vi "timerRun.vi"() -> ()   [LabVIEW 2012]
panel:
  in  "stop":bool
  out "Run time":timestamp
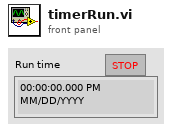
[diagram p1: front panel]
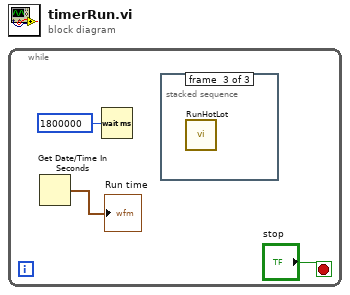
[diagram p0: block diagram]
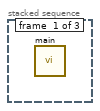
[diagram p2: hidden frame]
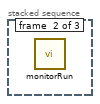
[diagram p3: hidden frame]
diagram:
  n1 = while {
    stop <- "stop" stop-if-true
    n2 = Get Date/Time In Seconds() -> (seconds since 1Jan1904=→"Run time":timestamp)
    n3 = Wait (ms)(milliseconds to wait=u32 1800000) -> ()  [unwired: 1 out]
    n4 = stacked-sequence {
      frame #0 {
        n5 = call "main.vi"() -> ()  [unwired: 10 in, 1 out]
      }
      frame #1 {
        n6 = call "monitorRun.vi"() -> ()  [unwired: 12 in]
      }
      frame #2 {
        n7 = call "RunHotLot.vi"() -> ()  [unwired: 12 in]
      }
    }
  }
